vi "OmniprobeFilter.vi"(8 "Probe Type":u16(ring)=12 items=["5-Hole Probe"=5, "OmniProbe"=12], 10 "ReductionCode":i32[](array[numeric]), 11 "RawVmagUVWCone":dbl[][](array[numeric]) caption="Raw\n   Vmag         U             V             W          Cone") -> (2 "FilteredVmagUVWCone":dbl[][](array[numeric]) caption="Filtered\n   Vmag          U               V              W        Cone")   [LabVIEW 2016]
uses:
  <vilib>/gmath/NI_Gmath.lvlib
  <vilib>/Analysis/NI_AALBase.lvlib
panel:
  in  "filterType":enum16{"SDclip", "Median"}(ring)
  in  "+/-Nsigma":dbl=3.0
  out "Stats-postfilter":dbl[][](array[numeric])
  out "Stats-prefilter":dbl[][](array[numeric])
  # "Mean"
  # "Var"
  # "Skew"
  # "Kurt"
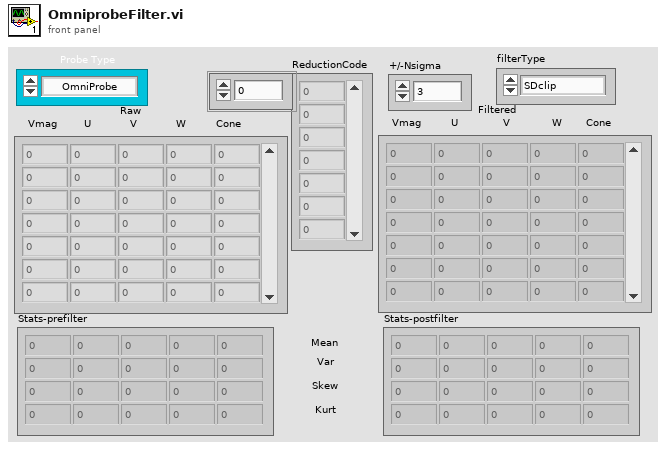
[diagram p1: front panel]
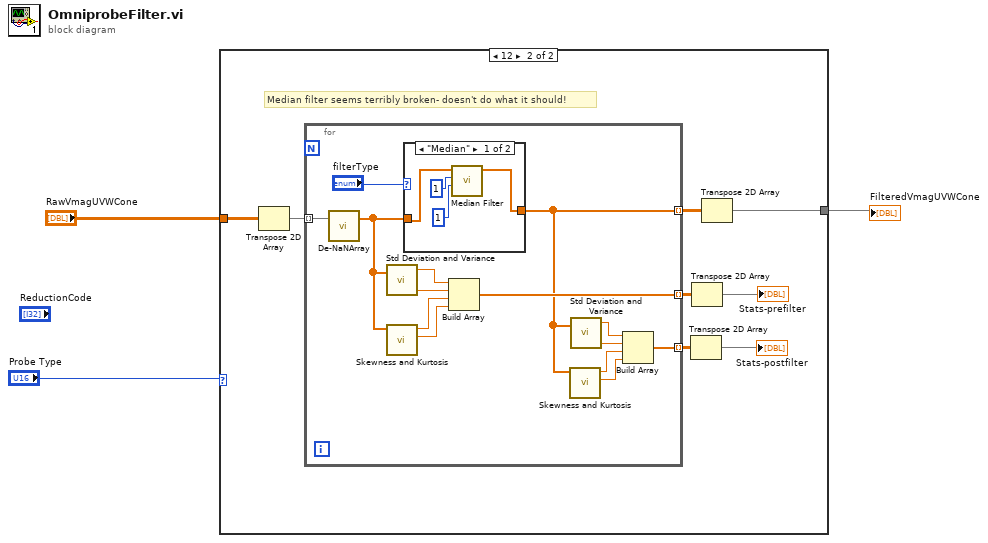
[diagram p0: block diagram]
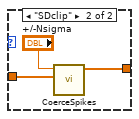
[diagram p3: hidden frame]
diagram:
  n1 = case shown="12" "Probe Type" {
    tunnel: "RawVmagUVWCone" -> [w4 w12]
    tunnel: [w4 w9] -> w2
    frame 5, Default {
    }
    frame 12 {
      # "Median filter seems terribly broken- doesn't do what it should!"
      n2 = Transpose 2D Array(2D array=w12) -> (transposed array=w10:dbl[][])
      n3 = for {
        tunnel: w10 -> [w18] mode=indexing
        tunnel: [w17] -> w11 mode=indexing
        tunnel: [w21] -> w8 mode=indexing
        tunnel: [w20] -> w7 mode=indexing
        n4 = call "De-NaNArray.vi"("ArrayIn"=w18) -> ("de-NaN-dArrayOut"=w16:dbl[])  [unwired: 1 in, 1 out]
        n5 = call <vilib>:"Std Deviation and Variance.vi"("X"=w16) -> ("mean"=w15:dbl, "variance"=w14:dbl)  [unwired: 1 in, 1 out]
        n6 = call <vilib>:"Skewness and Kurtosis.vi"("X"=w16) -> ("kurtosis"=w25:dbl, "skewness"=w26:dbl)  [unwired: 8 in, 1 out]
        n7 = case shown="\"Median\"" "filterType" {
          tunnel: [w29 w33] -> w17
          tunnel: w16 -> [w30 w31]
          frame "Median" {
            n8 = call <vilib>:"Median Filter.vi"("right rank"=1, "left rank"=1, "X"=w30) -> ("Filtered X"=w29:dbl[])  [unwired: 7 in, 1 out]
          }
          frame "SDclip" {
            n9 = call "CoerceSpikes.vi"("spikyData"=w31, "+/-Nsigma"="+/-Nsigma") -> ("deSpikedData"=w33:dbl[])  [unwired: 6 in, 3 out]
          }
        }
        n10 = Build Array(w15, w14, w26, w25) -> (w21:dbl[])
        n11 = call <vilib>:"Skewness and Kurtosis.vi"("X"=w17) -> ("kurtosis"=w24:dbl, "skewness"=w23:dbl)  [unwired: 8 in, 1 out]
        n12 = call <vilib>:"Std Deviation and Variance.vi"("X"=w17) -> ("mean"=w19:dbl, "variance"=w22:dbl)  [unwired: 1 in, 1 out]
        n13 = Build Array(w19, w22, w23, w24) -> (w20:dbl[])
      }
      n14 = Transpose 2D Array(2D array=w7) -> (transposed array=→"Stats-postfilter":dbl[][])
      n15 = Transpose 2D Array(2D array=w8) -> (transposed array=→"Stats-prefilter":dbl[][])
      n16 = Transpose 2D Array(2D array=w11) -> (transposed array=w9:dbl[][])
    }
  }
  "FilteredVmagUVWCone" <- w2
